vi "RG Fetch Waveform (Waveform Data Type) Split Channels.vi"(7 "error in (no error)":errorcluster, 8 "Maximum Time (10000ms)":u32=10000, 9 "Channel (0: Channel 1)":u16(ring) items=["Channel 1", "Channel 2", "Channel 3", "Channel 4", "Math", "Reference 1", "Reference 2", "Reference 3", "Reference 4", "D0", "D1", "D2", "D3", "D4", "D5", "D6", "D7", "D8", "D9", "D10", "D11", "D12", "D13", "D14", "D15", "Amplitude", "Frequency", "Phase", "Normal", "Average", "Maximum Peak Hold", "Minimum Peak Hold"], 10 "VISA resource name":refnum<visa-resource-name>) -> (0 "error out":errorcluster, 1 "Channel 2":dynamicdata(graph), 2 "Channel 1":dynamicdata(graph), 3 "VISA resource name out":refnum<visa-resource-name>)   [LabVIEW 2017, in "Scope.lvlib" / "Tektronix DPO MSO 2000 4000 Series.lvlib"]
doc: "Returns the waveform that an oscilloscope acquires for a channel you specify. An acquisition that you initiate before calling this VI generates the waveform.\n\nYou first enable channels with the Configure Channel VI. Then you use the Initiate VI to start an acquisition on the enabled channels. An oscilloscope concurrently acquires waveforms for these channels. You must call the Fetch Waveform VI separately to obtain waveforms for each enabled channel.\nHowever, you also can call the Read Waveform VI instead of using the above low-level VIs.\n\n<B>Note</B>: Use the Fetch Waveform VI only with other low-level VIs, such as the Initiate VI, the Abort VI, and the Fetch Waveform Measurement VI. High-level VIs, such as the Read Waveform VI, automatically incorporate the functions of the Initiate VI and the Fetch Waveform VI. The Fetch Waveform VI does not check the status of an instrument."
uses:
  Tektronix DPO MSO 2000 4000 Series.lvlib
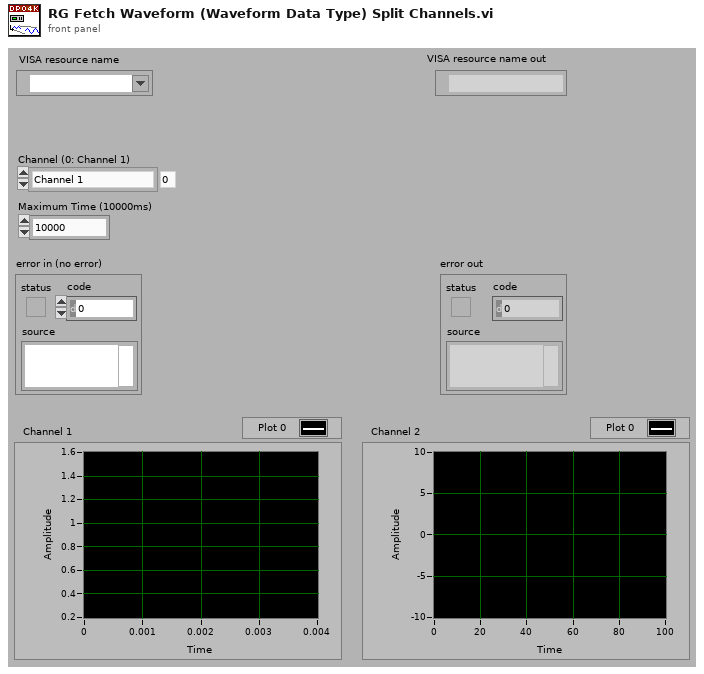
[diagram p1: front panel]
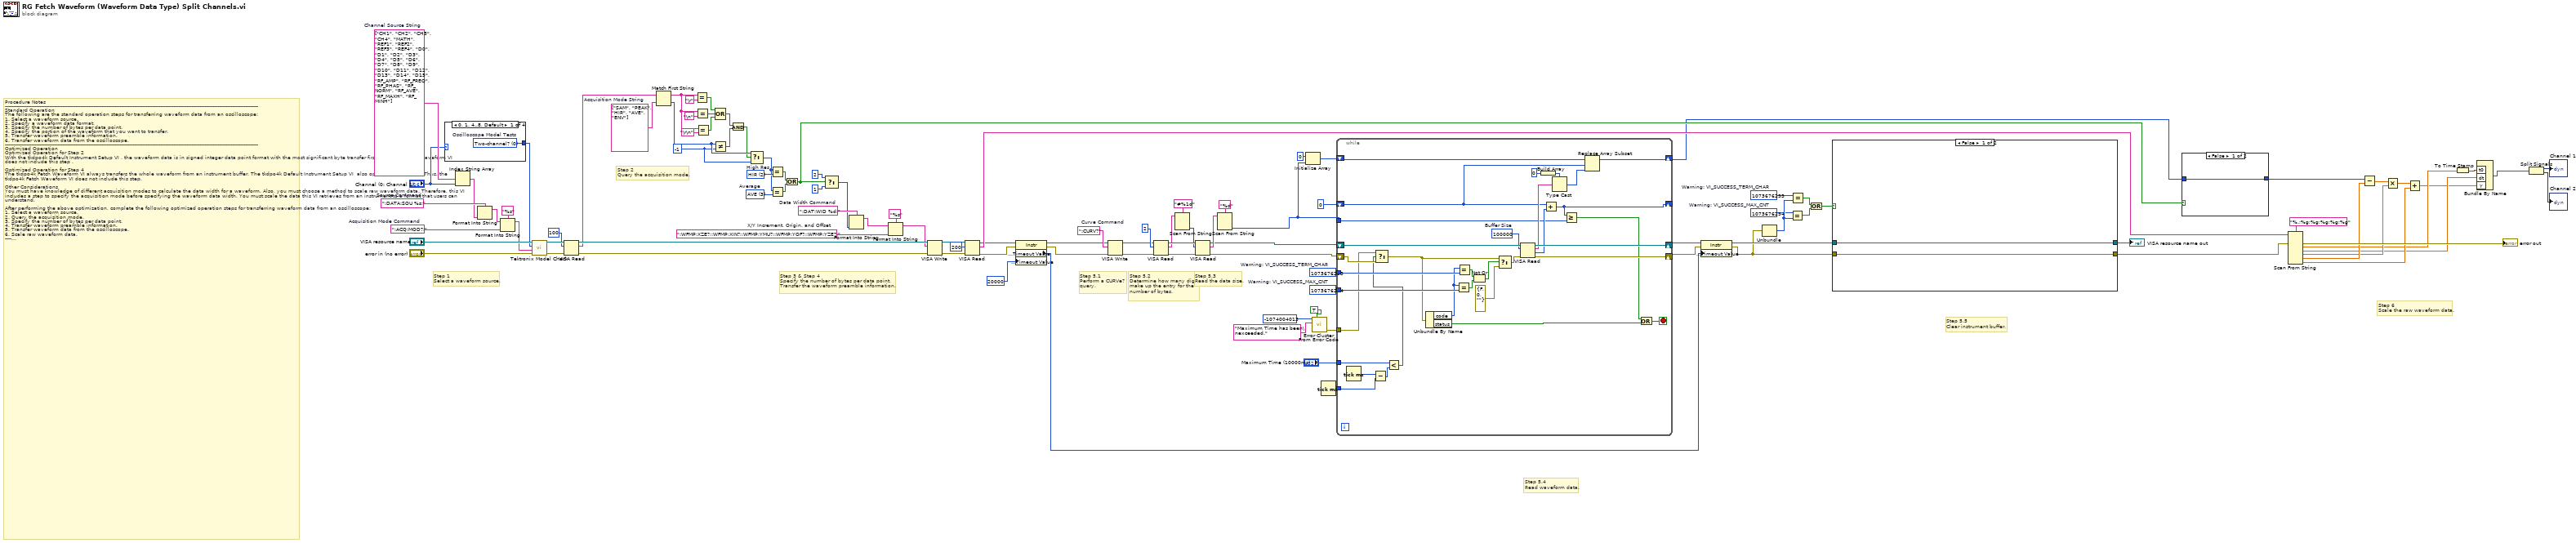
[diagram p0: block diagram]
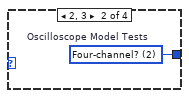
[diagram p2: hidden frame]
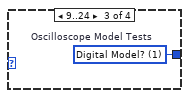
[diagram p3: hidden frame]
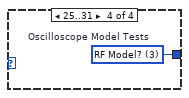
[diagram p4: hidden frame]
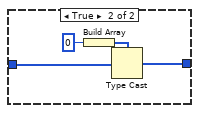
[diagram p5: hidden frame]
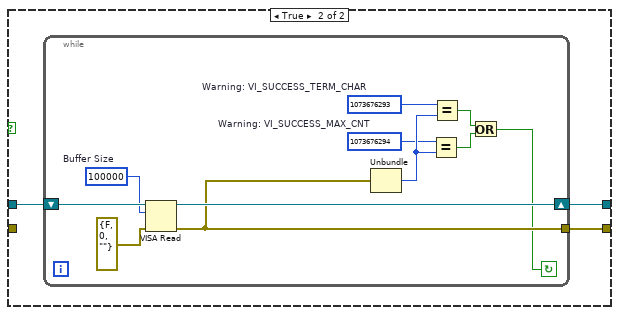
[diagram p6: hidden frame]
diagram:
  w46 = 1073676294  # Warning: VI_SUCCESS_MAX_CNT
  w47 = 1073676293  # Warning: VI_SUCCESS_TERM_CHAR
  w50 = 1073676294  # Warning: VI_SUCCESS_MAX_CNT
  w49 = 1073676293  # Warning: VI_SUCCESS_TERM_CHAR
  w59 = -1 ("y")
  w86 = ":CURV?"  # Curve Command
  w96 = ":DAT:WID %d;"  # Data Width Command
  w101 = u16 3 items=["SAM", "PEAK", "HIR", "AVE", "ENV"]  # Average
  w102 = u16 2 items=["SAM", "PEAK", "HIR", "AVE", "ENV"]  # High Res
  w71 = string[] ["SAM", "PEAK", "HIR", "AVE", "ENV"]  # Acquisition Mode String
  w95 = ":ACQ:MOD?;"  # Acquisition Mode Command
  w107 = string[] ["CH1", "CH2", "CH3", "CH4", "MATH", "REF1", "REF2", "REF3", "REF4", "D0", "D1", "D2", "D3", "D4", "D5", "D6", "D7", "D8", "D9", "D10", "D11", "D12", "D13", "D14", "D15", "RF_AMP", "RF_FREQ", "RF_PHAS", "RF_NORM", "RF_AVE", "RF_MAXH", "RF_MINH"]  # Channel Source String
  w106 = ":DATA:SOU %s;"  # Source Command
  w93 = ":WFMP:XZE?;:WFMP:XIN?;:WFMP:YMU?;:WFMP:YOF?;:WFMP:YZE?;"  # X/Y Increment, Origin, and Offset
  # "Step 6    \nScale the raw waveform data."
  # "Step 5.5    \nClear instrument buffer."
  # "Step 5.4   \nRead waveform data."
  # "Step 5.3      \nRead the data size."
  # "Step 5.2      \nDetermine how many digits\nmake up the entry for the \nnumber of bytes."
  # "Step 5.1      \nPerform a CURVe?\nquery."
  # "Step 3 & Step 4         \nSpecify the number of bytes per data point.\nTransfer the waveform preamble information."
  # "Step 2        \nQuery the acquisition mode."
  # "Step 1 \nSelect a waveform source."
  # "Procedure Notes\n-----------------------------------------------------------------------------------------------------------------------------------------------------------\nStandard Operation\nThe following are the standard operation steps for transferring waveform data from an oscilloscope:\n1. Select a waveform source.\n2. Specify a waveform data format.\n3. Specify the number of bytes per data point.\n4. Specify the portion of the waveform that you want to transfer.\n5. Transfer waveform preamble information.\n6. Transfer waveform data from the oscilloscope.\n-----------------------------------------------------------------------------------------------------------------------------------------------------------\nOptimized Operation\nOptimized Operation for Step 2\nWith the tkdpo4k Default Instrument Setup VI , the waveform data is in signed integer data point format with the most significant byte transfer first. Thus, the Fetch Waveform VI does not include this step . \n\nOptimized Operation for Step 4 \nThe tkdpo4k Fetch Waveform VI always transfers the whole waveform from an instrument buffer. The tkdpo4k Default Instrument Setup VI  also operates in this way. Thus, the tkdpo4k Fetch Waveform VI does not include this step. \n\nOther Considerations\nYou must have knowledge of different acquisition modes to calculate the data width for a waveform. Also, you must choose a method to scale raw waveform data. Therefore, this VI includes a step to specify the acquisition mode before specifying the waveform data width. You must scale the data this VI retrieves from an instrument to a format that users can understand.\n\nAfter performing the above optimization, complete the following optimized operation steps for transferring waveform data from an oscilloscope:\n1. Select a waveform source.\n2. Query the acquisition mode.\n3. Specify the number of bytes per data point.\n4. Transfer waveform preamble information.\n5. Transfer waveform data from the oscilloscope.\n6. Scale raw waveform data.\n-----------------------------------------------------------------------------------------------------------------------------------------------------------\nDetailed Steps\nThe following steps detail the behavior of this VI:\n1. Select a waveform source. \n2. Query and determine the acquisition mode. A correct determination is critical to steps 3 and 6.\n    -----------------------------------------------\n    Acquisition Mode |  Data Width   \n    -----------------------------------------------\n    Normal                       |   1                      \n    -----------------------------------------------\n    Peak Detect               |   1                      \n    -----------------------------------------------\n    Hi Res                        |   2                      \n    -----------------------------------------------\n    Envelope                   |   1                      \n    ----------------------------------------------- \n    Average                    |   2                      \n    -----------------------------------------------\n3. Specify the number of bytes per data point. For the Hi Res or Average acquisition modes, set the data width to 2. For all other acquisition modes, set the data width to 1.\n4. Transfer the waveform preamble information. Necessary preamble information includes XZero, XIncrement, YMultiplier, YOffset, and YZero. This VI uses XZero and XIncrement to configure the x-axis of output waveforms and uses YMultiplier, YOffset, and YZero to scale data values. This VI then parses the return string of the preamble query in step 6.\n5. Transfer waveform data from the oscilloscope.\n    5.1 Perform a CURVe? query.\n    5.2 Determine how many digits make up the entry for the number of bytes.\n    5.3 Read the data size.\n    5.4 Call the VISA Read VI repeatedly with a buffer size of 10000 until you obtain as much data as the data size specifies. Use      an 8-bit array to store the raw waveform data you obtain. \n    5.5 Continue reading the data remaining in the instrument buffer until the buffer is empty.\n6. Scale the raw waveform data.\n    6.1 Cast the waveform data to a 16-bit array if the data width is 2 . Split the waveform data into a minimum and a maximum data array if the acquisition mode is Peak Detect or Envelope. This VI skips this step if the data width is 1.\n    6.2 Parse the preamble information.\n    6.3 Scale the waveform data according to the following formula:\n          Data_Value_in_units = (Raw_Data_Value - YOffset) * YMultiplier + YZero\n          The resulting waveform data has a unit of volts.\n    6.4 Build a waveform graph."
  n1 = case shown="0, 1, 4..8, Default" "Channel (0: Channel 1)" {
    tunnel: [w108 w109 w110 w111] -> w4
    frame 0, 1, 4..8, Default {
      w108 = u16 0 items=["Two-channel?", "Digital Model?", "Four-channel?", "RF Model?"]  # Oscilloscope Model Tests
    }
    frame 2, 3 {
      w109 = u16 2 items=["Two-channel?", "Digital Model?", "Four-channel?", "RF Model?"]  # Oscilloscope Model Tests
    }
    frame 9..24 {
      w110 = u16 1 items=["Two-channel?", "Digital Model?", "Four-channel?", "RF Model?"]  # Oscilloscope Model Tests
    }
    frame 25..31 {
      w111 = u16 3 items=["Two-channel?", "Digital Model?", "Four-channel?", "RF Model?"]  # Oscilloscope Model Tests
    }
  }
  n2 = Index String Array(1:"Channel (0: Channel 1)", 2:w107) -> (0:w105:string)  [unwired: 1 in]
  n3 = Format Into String(format string=w106, w105) -> (resulting string=w104:string)  [unwired: 2 in, 1 out]
  n4 = Format Into String(format string="%s", initial string=w104, w95) -> (resulting string=w9:string)  [unwired: 1 in, 1 out]
  n5 = call "Tektronix Model Check.vi"("error in (no error)"="error in (no error)", "Command String"=w9, "Oscilloscope Model Tests (3: RF Model?)"=w4, "VISA resource name"="VISA resource name") -> ("error out"=w7:errorcluster, "VISA resource name out"=w8:refnum<visa-resource-name>)  [unwired: 6 in]
  n6 = VISA Read(VISA resource name=w8, byte count=u32 100, error in (no error)=w7) -> (VISA resource name out=w92:refnum<visa-resource-name>, read buffer=w70:string, error out=w91:errorcluster)  [unwired: 1 out]
  n7 = Match First String(2:w71, 3:w70) -> (0:w60:i32, 1:w66:string)
  n8 = Equal?(x=w66, y="\r") -> (x = y?=w65:bool)
  n9 = Equal?(x=w66, y="\n") -> (x = y?=w64:bool)
  n10 = Equal?(x=w66, y="\r\n") -> (x = y?=w63:bool)
  n11 = Not Equal?(x=w60, y=w59) -> (x != y?=w61:bool)
  n12 = Compound Arithmetic op=OR(w65, w64, w63) -> (w62:bool)
  n13 = And(x=w62, y=w61) -> (x .and. y?=w58:bool)
  n14 = Select(t=w60, s=w58, f=w59) -> (s? t:f=w45:i32)
  n15 = Equal?(x=w45, y=w102) -> (x = y?=w100:bool)
  n16 = Equal?(x=w45, y=w101) -> (x = y?=w99:bool)
  n17 = Or(x=w100, y=w99) -> (x .or. y?=w44:bool)
  n18 = Select(t=2 ("f"), s=w44, f=1) -> (s? t:f=w76:i32)
  n19 = Format Into String(format string=w96, w76) -> (resulting string=w90:string)  [unwired: 2 in, 1 out]
  n20 = Format Into String(format string="%s", initial string=w90, w93) -> (resulting string=w77:string)  [unwired: 1 in, 1 out]
  n21 = VISA Write(VISA resource name=w92, write buffer=w77, error in (no error)=w91) -> (VISA resource name out=w88:refnum<visa-resource-name>, error out=w87:errorcluster)  [unwired: 1 out]
  n22 = VISA Read(VISA resource name=w88, byte count=u32 200, error in (no error)=w87) -> (VISA resource name out=w19:refnum<visa-resource-name>, read buffer=w75:string, error out=w18:errorcluster)  [unwired: 1 out]
  n23 = property class="Instr"(reference=w19, error in=w18, "General Settings:Timeout Value"=u32 20000) -> (reference out=w17:refnum<visa-resource-name>, error out=w15:errorcluster, "General Settings:Timeout Value"=w28:u32)
  n24 = VISA Write(VISA resource name=w17, write buffer=w86, error in (no error)=w15) -> (VISA resource name out=w16:refnum<visa-resource-name>, error out=w14:errorcluster)  [unwired: 1 out]
  n25 = VISA Read(VISA resource name=w16, byte count=u32 2, error in (no error)=w14) -> (VISA resource name out=w83:refnum<visa-resource-name>, read buffer=w81:string, error out=w82:errorcluster)  [unwired: 1 out]
  n26 = Scan From String(format string="#%1d", input string=w81) -> (output 1=w80:i32)  [unwired: 3 in, 3 out]
  n27 = VISA Read(VISA resource name=w83, byte count=w80, error in (no error)=w82) -> (VISA resource name out=w13:refnum<visa-resource-name>, read buffer=w78:string, error out=w12:errorcluster)  [unwired: 1 out]
  n28 = Scan From String(format string="%d", input string=w78) -> (output 1=w57:i32)  [unwired: 3 in, 3 out]
  n29 = Initialize Array(i8 0 ("element"), w57) -> (w55:i8[])
  n30 = call <vilib>:"Error Cluster From Error Code.vi"("show call chain? (False)"=TRUE, "error message (\"\")"="Maximum Time has been\nexceeded." ("error message (\"\")"), "error code (0)"=-1074004013) -> ("error out"=w20:errorcluster)  [unwired: 6 in]
  n31 = Tick Count (ms)() -> (millisecond timer value=w25:u32)
  n32 = while {
    shift-right: [w142] -> w30
    shift-left: w13 -> [w144]
    shift-right: [w141] -> w29
    shift-left: w12 -> [w114]
    shift-right: [w137] -> w43
    shift-left: w55 -> [w138]
    tunnel: w57 -> [w134]
    shift-right: [w131] -> _
    shift-left: 0 -> [w132]
    tunnel: w47 -> [w125]
    tunnel: w46 -> [w124]
    tunnel: w25 -> [w118]
    tunnel: "Maximum Time (10000ms)" -> [w116]
    tunnel: w20 -> [w113]
    stop <- w130 stop-if-true
    w143 = 100000  # Buffer Size
    n33 = Tick Count (ms)() -> (millisecond timer value=w119:u32)
    n34 = Subtract(x=w119, y=w118) -> (x-y=w117:u32)
    n35 = Less?(x=w116, y=w117) -> (x < y?=w112:bool)
    n36 = Select(t=w113, s=w112, f=w114) -> (s? t:f=w115:errorcluster)
    n37 = Unbundle By Name(w115) -> ("code"=w123:i32, "status"=w127:bool)
    n38 = Equal?(x=w123, y=w124) -> (x = y?=w121:bool)
    n39 = Equal?(x=w123, y=w125) -> (x = y?=w122:bool)
    n40 = Not Or(1:w121, 2:w122) -> (0:w120:bool)
    n41 = Select(t=w115, s=w120, f=errorcluster {"status"=FALSE, "code"=0, "source"=""} ("error in (no error)")) -> (s? t:f=w126:errorcluster)
    n42 = VISA Read(VISA resource name=w144, byte count=w143, error in (no error)=w126) -> (VISA resource name out=w142:refnum<visa-resource-name>, read buffer=w136:string, return count=w135:u32, error out=w141:errorcluster)
    n43 = Build Array(i8 0) -> (w140:i8[])
    n44 = Add(x=w132, y=w135) -> (x+y=w131:u32)
    n45 = Type Cast(type=w140, x=w136) -> (*(type *) &x=w133:i8[])
    n46 = Greater Or Equal?(x=w131, y=w134) -> (x >= y?=w129:bool)
    n47 = Replace Array Subset(array=w138, new element=w133, index=w132) -> (w137:i8[])
    n48 = Compound Arithmetic op=OR(w129, w127) -> (w130:bool)
  }
  n49 = property class="Instr"(reference=w30, error in=w29, "General Settings:Timeout Value"=w28) -> (reference out=w27:refnum<visa-resource-name>, error out=w26:errorcluster)
  n50 = Unbundle(w26) -> ("code"=w51:i32)  [unwired: 2 out]
  n51 = Equal?(x=w50, y=w51) -> (x = y?=w53:bool)
  n52 = Equal?(x=w49, y=w51) -> (x = y?=w54:bool)
  n53 = Or(x=w54, y=w53) -> (x .or. y?=w52:bool)
  n54 = case shown="False" w52 {
    tunnel: w27 -> [w146 w149]
    tunnel: w26 -> [w145 _]
    tunnel: [w146 w148] -> w72
    tunnel: [w145 w147] -> w74
    frame False {
    }
    frame True {
      n55 = while {
        shift-right: [w159] -> w148
        shift-left: w149 -> [w160]
        tunnel: [w152] -> w147
        stop <- w151 continue-if-true
        w154 = 1073676294  # Warning: VI_SUCCESS_MAX_CNT
        w153 = 1073676293  # Warning: VI_SUCCESS_TERM_CHAR
        w158 = u32 100000  # Buffer Size
        n56 = VISA Read(VISA resource name=w160, byte count=w158, error in (no error)=errorcluster {"status"=FALSE, "code"=0, "source"=""}) -> (VISA resource name out=w159:refnum<visa-resource-name>, error out=w152:errorcluster)  [unwired: 2 out]
        n57 = Unbundle(w152) -> ("code"=w155:i32)  [unwired: 2 out]
        n58 = Equal?(x=w154, y=w155) -> (x = y?=w156:bool)
        n59 = Equal?(x=w153, y=w155) -> (x = y?=w157:bool)
        n60 = Or(x=w157, y=w156) -> (x .or. y?=w151:bool)
      }
    }
  }
  "VISA resource name out" <- w72
  n61 = case shown="False" w44 {
    tunnel: w43 -> [w161 w163]
    tunnel: [w161 w162] -> w32
    frame False {
    }
    frame True {
      n62 = Build Array(i16 0 ("element")) -> (w164:i16[])
      n63 = Type Cast(type=w164, x=w163) -> (*(type *) &x=w162:i16[])
    }
  }
  n64 = Scan From String(format string="%.;%g;%g;%g;%g;%g", input string=w75, error in=w74) -> (error out=→"error out":errorcluster, output 1=w36:dbl, output 2=w35:dbl, output 3=w37:dbl, output 4=w38:dbl, output 5=w39:dbl)  [unwired: 6 in, 2 out]
  n65 = Subtract(x=w32, y=w38) -> (x-y=w41:dbl[])
  n66 = Multiply(x=w41, y=w37) -> (x*y=w40:dbl[])
  n67 = Add(x=w40, y=w39) -> (x+y=w34:dbl[])
  n68 = To Time Stamp(1:w36) -> (0:w33:timestamp)
  n69 = Bundle By Name("t0"=w33, "dt"=w35, "Y"=w34) -> (w3:waveform(dbl))  [unwired: 1 in]
  n70 = Split Signals(w3) -> (→"Channel 1":dynamicdata, →"Channel 2":dynamicdata)  [unwired: 2 in]
